vi "ADstar with maping inline.vi"() -> ()   [LabVIEW 2012]
doc: "This example continually replans a path from Start to Goal while following the best known path, including through obstacles if necessary.\nThe Anytime D* search algorithm is useful when the world or the robot's understanding of the world is changing. Anytime D* maintains more information than the A* search algorithm so the robot can backtrack and find a new path more easily if it discovers the original path will not work."
uses:
  <vilib>/robotics/Navigation/shared/WorldMap/OccupancyGridWorldMap/NI_Robotics_OccupancyGridWorldMap.lvclass
  <vilib>/robotics/Navigation/Anytime D Star/NI_Robotics_AnytimeDStar.lvclass
panel:
  in  "Rotation (deg)":i32
  in  "Y displacement":i32
  in  "X dispacement":i32
  in  "Step Through":bool
  in  "goal y":i32=49
  in  "goal x":i32=49
  out "Open List Size":i32(graph)=1665
  out "path on obstacles":dbl[][](graph)
  out "AD* Open Nodes":i32=1665 caption="size"
  out "Path Cost":dbl(graph)
  in  "Epsilon":i32=2 min=1
  out "AD* Path Cost":dbl caption="path cost"
  in  "y start":i32
  in  "x start":i32
  in  "Move Robot":i32=1 min=0
  in  "Overhaul":i32=25
  in  "step button":bool
  out "AD* Time":u32=117 caption="seconds"
  out "Compute Path Time":u32(graph)=117
  in  "stop":bool
  # "The Anytime D* search algorithm is useful when the world or the robot's understanding of the world is changing.  Anytime D* maintains more information\n than the A* search algorithm so the robot can backtrack and find a new path more easily if it discovers the original path will not work."
  # "This example continually replans a path from Start to Goal while \nfollowing the best known path, including through obstacles if necessary."
  # "Configuration"
  # "X"
  # "Y"
  # "Start"
  # "Goal"
  # "Run Mode"
  # "Run-time Control"
  # "Detection radius of robot's sensors."
  # "Number of steps the robot takes after each plan."
  # "Number of steps before AD* plans from scratch."
  # "1) Choose the Start and Goal location and the % Random Obstacles.\n2) Run the VI.\n3) Adjust the controls in the Run-time Controls section to see the \n     effect each option has on path planning\n4) Change the Run Mode to Single Step to pause after each time\n the AD* VI runs"
  # "A higher epsilon results in a faster but less optimal search."
  # "Continuous"
  # "Single Step"
  # "Robot"
  # "Obstacle"
  # "Unknown"
  # "Free"
  # "Path"
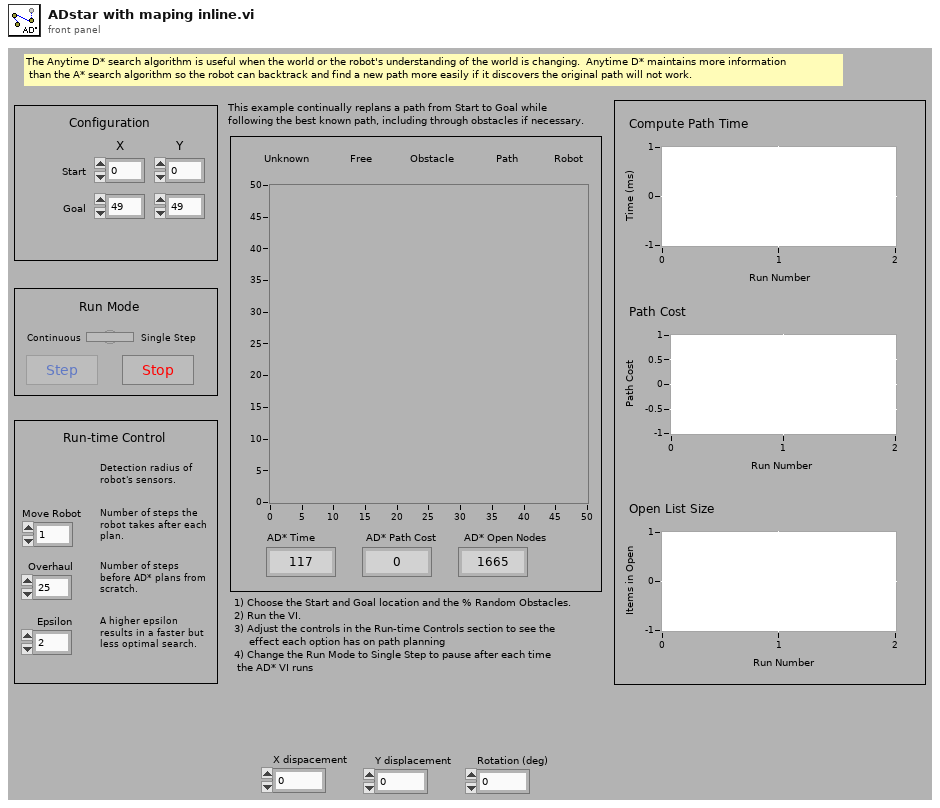
[diagram p1: front panel]
types:
  T1 = enum8{"Enabled", "Disabled", "Disabled and Grayed Out"}
  T2 = cluster{"epsilon":dbl, "run number":i32, "open list size":i32}
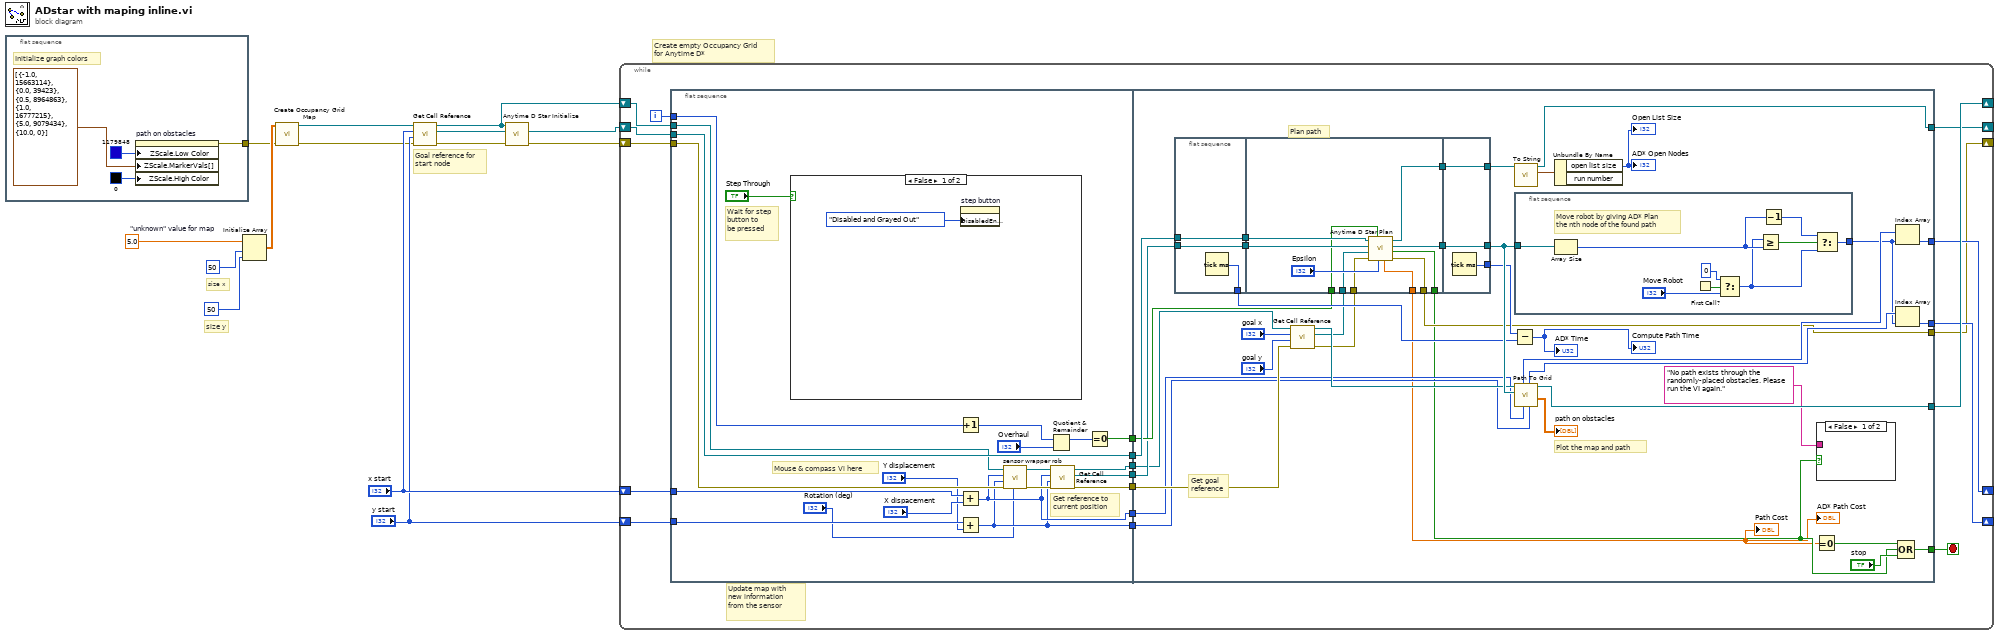
[diagram p0: block diagram]
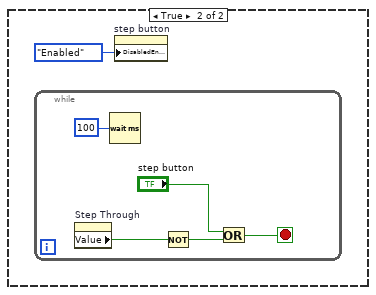
[diagram p2: hidden frame]
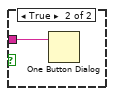
[diagram p3: hidden frame]
diagram:
  w12 = 5.0  # "unknown" value for map
  # "Goal reference for\nstart node"
  # "size y"
  # "size x"
  # "Create empty Occupancy Grid\nfor Anytime D*"
  n1 = flat-sequence {
    tunnel: [w15] -> w5
    frame #0 {
      # "Initialize graph colors"
      n2 = property on="path on obstacles" class="IntGraph (strict)"("ZScale.Low Color"=u32 1179848, "ZScale.MarkerVals[]"=cluster{dbl, u32}[] [{-1.0, 15663114}, {0.0, 39423}, {0.5, 8964863}, {1.0, 16777215}, {5.0, 9079434}, {10.0, 0}], "ZScale.High Color"=u32 0) -> (error out=w15:errorcluster)  [unwired: 2 in, 1 out]
    }
  }
  n3 = Initialize Array(w12, 50 ("y"), 50 ("x")) -> (w9:dbl[][])
  n4 = call <vilib>:"Create Occupancy Grid Map.vi"("error in (no error)"=w5, "occupancy grid"=w9) -> ("error out"=w7:errorcluster, "map reference out"=w2:refnum<data-value>)  [unwired: 8 in]
  n5 = call <vilib>:"Get Cell Reference.vi"("error in (no error)"=w7, "y"="y start", "x"="x start", "map reference in"=w2) -> ("error out"=w6:errorcluster, "cell reference"=w8:refnum<data-value>, "map reference out"=w3:refnum<data-value>)  [unwired: 4 in, 1 out]
  n6 = call <vilib>:"Anytime D Star Initialize.vi"("error in (no error)"=w6, "start reference"=w8, "map reference in"=w3) -> ("error out"=w1:errorcluster, "Anytime D*"=w4:refnum<class "NI_Robotics_AnytimeDStar.lvclass">)  [unwired: 7 in]
  n7 = while {
    shift-right: [w32] -> _
    shift-left: w4 -> [w37]
    shift-right: [w36] -> _
    shift-left: w3 -> [w22]
    shift-right: [w31] -> _
    shift-left: "x start" -> [w19]
    shift-right: [w30] -> _
    shift-left: "y start" -> [w20]
    shift-right: [w26] -> _
    shift-left: w1 -> [w21]
    i -> [w29]
    stop <- w23 stop-if-true
    # "Update map with new information\nfrom the sensor"
    n8 = flat-sequence {
      tunnel: w29 -> [w51]
      tunnel: w22 -> [w48]
      tunnel: w37 -> [w58]
      tunnel: [w58] -> w35
      tunnel: [w57] -> w34
      tunnel: [w56] -> w33
      tunnel: w19 -> [w43]
      tunnel: w20 -> [w41]
      tunnel: [w50] -> w28
      tunnel: w21 -> [w45]
      tunnel: [w49] -> w27
      tunnel: [w42] -> w25
      tunnel: [w39] -> w24
      tunnel: [w68] -> w23
      tunnel: [w102] -> w32
      tunnel: [w90] -> w36
      tunnel: [w83] -> w31
      tunnel: [w82] -> w30
      tunnel: w28 -> [w88]
      tunnel: w33 -> [w87]
      tunnel: w34 -> [w81]
      tunnel: w35 -> [w98]
      tunnel: w27 -> [w78]
      tunnel: [w74] -> w26
      tunnel: w25 -> [w73]
      tunnel: w24 -> [w72]
      frame #0 {
        # "Mouse & compass Vi here"
        # "Get reference to \ncurrent position"
        # "Wait for step\nbutton to\nbe pressed"
        n9 = case shown="False" "Step Through" {
          frame False {
            n10 = property on="step button" class="Bool"("DisabledEnum"=T1."Disabled and Grayed Out" ("Disabled")) -> ()  [unwired: 2 in, 2 out]
          }
          frame True {
            n11 = while {
              stop <- w63 stop-if-true
              n12 = property on="Step Through" class="Bool (strict)"() -> ("Value"=w61:bool)  [unwired: 2 in, 2 out]
              n13 = Wait (ms)(milliseconds to wait=u32 100) -> ()  [unwired: 1 out]
              n14 = Not(x=w61) -> (.not. x?=w62:bool)
              n15 = Or(x="step button", y=w62) -> (x .or. y?=w63:bool)
            }
            n16 = property on="step button" class="Bool"("DisabledEnum"=T1."Enabled" ("Disabled")) -> ()  [unwired: 2 in, 2 out]
          }
        }
        n17 = Increment(x=w51) -> (x+1=w53:i32)
        n18 = Add(x=w43, y="X dispacement") -> (x+y=w42:i32)
        n19 = Add(x=w41, y="Y displacement") -> (x+y=w39:i32)
        n20 = call "sensor wrapper rob.vi"("Degrees"="Rotation (deg)", "error in (no error)"=w45, "sensor y"=w39, "Sensor x"=w42, "map reference in"=w48) -> ("error out"=w46:errorcluster, "map reference out 2"=w47:refnum<data-value>)  [unwired: 5 in]
        n21 = Quotient & Remainder(x=w53, y="Overhaul") -> (x-y*floor(x/y)=w52:i32)  [unwired: 1 out]
        n22 = call <vilib>:"Get Cell Reference.vi"("error in (no error)"=w46, "y"=w39, "x"=w42, "map reference in"=w47) -> ("error out"=w49:errorcluster, "cell reference"=w56:refnum<data-value>, "map reference out"=w57:refnum<data-value>)  [unwired: 4 in, 1 out]
        n23 = Equal To 0?(x=w52) -> (x = 0?=w50:bool)
      }
      frame #1 {
        # "Plot the map and path"
        # "Get goal \nreference"
        # "Plan path"
        n24 = flat-sequence {
          tunnel: w98 -> [w115]
          tunnel: w87 -> [w116]
          tunnel: [w116] -> w97
          tunnel: [w115] -> w96
          tunnel: [w114] -> w92
          tunnel: [w123] -> w69
          tunnel: [w122] -> w67
          tunnel: w97 -> [w126]
          tunnel: w96 -> [w127]
          tunnel: [w124] -> w95
          tunnel: [w125] -> w94
          tunnel: w88 -> [w120]
          tunnel: w76 -> [w119]
          tunnel: w75 -> [w118]
          tunnel: [w117] -> w74
          tunnel: [w129] -> w101
          tunnel: [w130] -> w103
          tunnel: w95 -> [w130]
          tunnel: w94 -> [w129]
          tunnel: [w128] -> w93
          frame #0 {
            n25 = Tick Count (ms)() -> (millisecond timer value=w114:u32)
          }
          frame #1 {
            n26 = call <vilib>:"Anytime D Star Plan.vi"("epsilon"="Epsilon", "overhaul (F)"=w120, "error in (no error)"=w118, "new goal reference"=w119, "current reference"=w126, "Anytime D* in"=w127) -> ("error out"=w117:errorcluster, "no valid path exists"=w123:bool, "path references"=w125:refnum<data-value>[], "Anytime D* out"=w124:refnum<class "NI_Robotics_AnytimeDStar.lvclass">, "path cost"=w122:dbl)  [unwired: 1 in]
          }
          frame #2 {
            n27 = Tick Count (ms)() -> (millisecond timer value=w128:u32)
          }
        }
        n28 = call <vilib>:"Get Cell Reference.vi"("error in (no error)"=w78, "y"="goal y", "x"="goal x", "map reference in"=w81) -> ("error out"=w75:errorcluster, "cell reference"=w76:refnum<data-value>, "map reference out"=w77:refnum<data-value>)  [unwired: 4 in, 1 out]
        n29 = Subtract(x=w93, y=w92) -> (x-y=→"Compute Path Time" →"AD* Time":u32)
        n30 = call <vilib>:"To String.vi"("Anytime D* in"=w103) -> ("output"=w100:T2, "Anytime D* out"=w102:refnum<class "NI_Robotics_AnytimeDStar.lvclass">)  [unwired: 8 in, 1 out]
        n31 = flat-sequence {
          tunnel: w101 -> [w112]
          tunnel: [w105] -> w84
          frame #0 {
            # "Move robot by giving AD* Plan\nthe nth node of the found path"
            n32 = Array Size(array=w112) -> (size(s)=w109:i32)
            n33 = First Call?() -> (First Call?: T/F=w111:bool)
            n34 = Select(t=0, s=w111, f="Move Robot") -> (s? t:f=w108:i32)
            n35 = Greater Or Equal?(x=w108, y=w109) -> (x >= y?=w107:bool)
            n36 = Decrement(x=w109) -> (x-1=w113:i32)
            n37 = Select(t=w113, s=w107, f=w108) -> (s? t:f=w105:i32)
          }
        }
        n38 = call "Path To Grid.vi"("current y"=w72, "current x"=w73, "path references"=w101, "map reference in"=w77) -> ("path on obstacles"=→"path on obstacles":dbl[][], "map reference out"=w90:refnum<data-value>, "y coordinates"=w86:i32[], "x coordinates"=w85:i32[])  [unwired: 3 in, 1 out]
        n39 = Unbundle By Name(w100) -> ("open list size"=→"Open List Size" →"AD* Open Nodes":i32)  [unwired: 1 out]
        n40 = Equal To 0?(x=w67) -> (x = 0?=w66:bool)
        n41 = case shown="False" w69 {
          tunnel: "No path exists through the randomly-placed obstacles. Please run the VI again." -> [_ w104]
          frame False {
          }
          frame True {
            n42 = One Button Dialog(message=w104) -> ()  [unwired: 1 in, 1 out]
          }
        }
        n43 = Index Array(array=w85, index=w84) -> (element=w83:i32)
        n44 = Index Array(array=w86, index=w84) -> (element=w82:i32)
        n45 = Compound Arithmetic op=OR(w66, w69, "stop") -> (w68:bool)
        "AD* Path Cost" <- w67
        "Path Cost" <- w67
      }
    }
  }
